vi "LOER Node Tester.vi"() -> ()   [LabVIEW 2016]
uses:
  <vilib>/LIEF/Image Editor Handler/Image Editor Handler.lvclass
  LIEF-Examples/LIEF Imager/Imager Editor Handler/Imager Handler.lvclass
  LOER XNode/LV Object Event Registration Node.xnode
  LIEF-Examples/LIEF Imager/Imager Editor Handler/Read SystemPropertyChanged Event.vi
  <vilib>/LIEF/Image Editor Handler/Read Events.vi
panel:
  out "class path":path
  out "class name":string
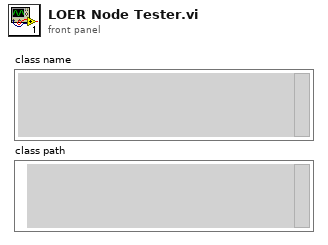
[diagram p1: front panel]
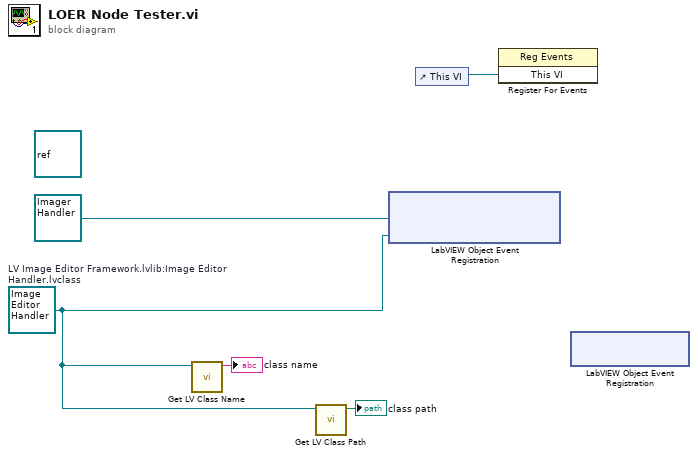
[diagram p0: block diagram]
diagram:
  (unwired) refnum<class> refnum ("LabVIEW Object")
  w1 = refnum<class "Image Editor Handler.lvclass"> refnum  # LV Image Editor Framework.lvlib:Image Editor Handler.lvclass
  n1 = call <vilib>:"Get LV Class Name.vi"("object"=w1) -> ("class name"=→"class name":string)  [unwired: 9 in, 1 out]
  n2 = call <vilib>:"Get LV Class Path.vi"("object"=w1) -> ("class path"=→"class path":path)  [unwired: 9 in, 1 out]
  n3 = xnode "LabVIEW Object Event Registration"("Object_1"=refnum<class "Imager Handler.lvclass"> refnum ("Imager Handler.lvclass"), "Object_2"=w1) -> ()  [unwired: 1 in, 2 out]
  n4 = control-ref of="This VI"() -> (w4:refnum<vi>)
  n5 = register-events(w4) -> ()  [unwired: 2 in, 2 out]
  n6 = xnode "LabVIEW Object Event Registration"() -> ()  [unwired: 2 in, 2 out]
